vi "FITS Update Header Field.vi"   [LabVIEW 2022 SP3]
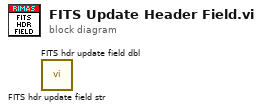
[diagram p0: block diagram]
diagram:
  n1 = call "FITS hdr update field str.vi"() -> ()  [unwired: 10 in, 2 out]
  n2 = call "FITS hdr update field dbl.vi"() -> ()  [unwired: 10 in, 2 out]
